vi "Test_IOVariable.vi"(8 "error in (no error)":errorcluster) -> (0 "error out":errorcluster)   [LabVIEW 2013]
uses:
  source/uri/URI.lvclass/URI.ctl
  source/components/path/URI-Component.Path.lvclass/URI-Component.Path.ctl
  source/uri/Read scheme.vi
  source/uri/Read host.vi
  source/uri/Read path.vi
  source/components/path/Get Segments.vi
  source/utilities/Percent-Encode String.vi
  source/utilities/isHEXDigit.vi
  <vilib>/addons/_JKI Toolkits/Caraya/classes/Assert/Assert Equal Value_Variant.vi
  <vilib>/addons/_JKI Toolkits/Caraya/classes/Assert/Assert True.vi
  source/components/path/Create Path (string).vi
  <vilib>/addons/_JKI Toolkits/Caraya/classes/Test/Test.lvclass
  <vilib>/addons/_JKI Toolkits/Caraya/classes/Assert/Assert.lvclass
  source/uri/URI.lvclass
  source/openURI.lvlib
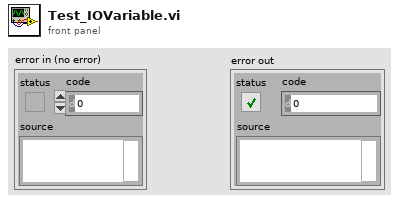
[diagram p1: front panel]
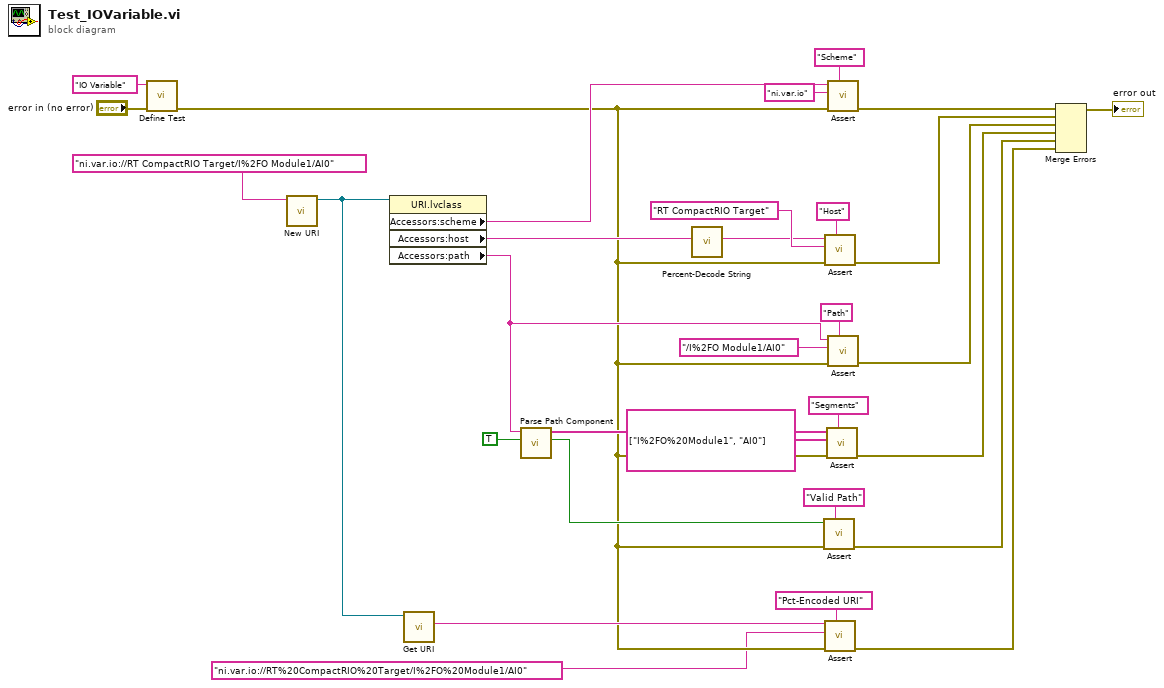
[diagram p0: block diagram]
diagram:
  n1 = call <vilib>:"Define Test.vi"("error in (no error)"="error in (no error)", "Label (VI Title)"="IO Variable") -> ("error out"=w3:errorcluster)  [unwired: 9 in]
  n2 = call "New URI.vi"("URI"="ni.var.io://RT CompactRIO Target/I%2FO Module1/AI0") -> ("URI"=w6:refnum<class "URI.lvclass">)  [unwired: 9 in, 1 out]
  n3 = property on="Property Node" class="URI.lvclass"(reference=w6) -> ("Accessors:scheme"=w26:string, "Accessors:host"=w10:string, "Accessors:path"=w8:string)  [unwired: 1 in, 2 out]
  n4 = call "Get URI.vi"("URI in"=w6) -> ("URI String"=w4:string)  [unwired: 8 in, 2 out]
  n5 = call "Parse Path Component.vi"("Pct-Encode (F)"=TRUE, "path"=w8) -> ("valid"=w14:bool, "Segments"=w16:string[])  [unwired: 8 in]
  n6 = call "Percent-Decode String.vi"("Pct-Encoded String"=w10) -> ("String"=w9:string)  [unwired: 10 in]
  n7 = call-poly <vilib>:"Assert.vi"("Label"="Valid Path" ("URI"), "error in (no error)"=w3, "True?"=w14) -> ("error out"=w12:errorcluster)  [unwired: 8 in]
  n8 = call-poly <vilib>:"Assert.vi"("Label"="Host" ("URI"), "error in (no error)"=w3, "Y"="RT CompactRIO Target" ("URI"), "X"=w9) -> ("error out"=w22:errorcluster)  [unwired: 7 in]
  n9 = call-poly <vilib>:"Assert.vi"("Label"="Pct-Encoded URI" ("URI"), "error in (no error)"=w3, "Y"="ni.var.io://RT%20CompactRIO%20Target/I%2FO%20Module1/AI0" ("URI"), "X"=w4) -> ("error out"=w2:errorcluster)  [unwired: 7 in]
  n10 = call-poly <vilib>:"Assert.vi"("Label"="Segments" ("URI"), "error in (no error)"=w3, "Y"=string[] ["I%2FO%20Module1", "AI0"] ("Segments"), "X"=w16) -> ("error out"=w15:errorcluster)  [unwired: 7 in]
  n11 = call-poly <vilib>:"Assert.vi"("Label"="Scheme" ("URI"), "error in (no error)"=w3, "Y"="ni.var.io" ("URI"), "X"=w26) -> ("error out"=w23:errorcluster)  [unwired: 7 in]
  n12 = call-poly <vilib>:"Assert.vi"("Label"="Path" ("URI"), "error in (no error)"=w3, "Y"="/I%2FO Module1/AI0" ("URI"), "X"=w8) -> ("error out"=w19:errorcluster)  [unwired: 7 in]
  n13 = Merge Errors(w23, w22, w19, w15, w12, w2) -> (→"error out":errorcluster)
